vi "Read Add Undo.vi"(8 "error in":errorcluster, 11 "History in":refnum<class "History.lvclass">) -> (0 "error out":errorcluster, 2 "Add Undo":bool, 3 "History out":refnum<class "History.lvclass">)   [LabVIEW 2020, in "lv_icon.lvlib" / "History.lvlib" / "History.lvclass"]
uses:
  History.lvclass
  History.lvclass/History.ctl
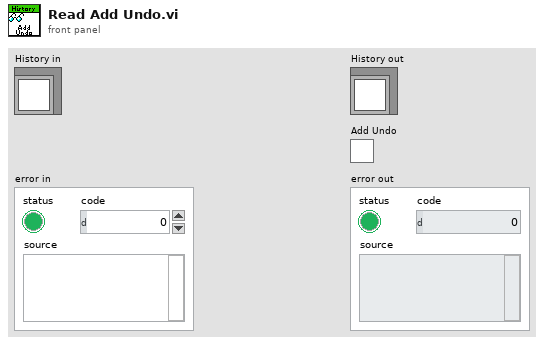
[diagram p1: front panel]
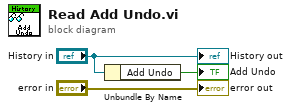
[diagram p0: block diagram]
diagram:
  n1 = Unbundle By Name("History in") -> ("Add Undo"=→"Add Undo":bool)
  "History out" <- "History in"
  "error out" <- "error in"
